vi "Timeout value.vi"(11 "Loop data in":T1={"Config"={"List"=[], "max rows"=8, "Listbox placement"=enum."None", "String Color Options"={"Use? (F)"=FALSE, "Color - Valid"=0, "Color - Invalid"=0, "Allow blank?"=FALSE}}, "Refs"={"String"=refnum, "Listbox"=refnum}, "State"={"LB active?"=FALSE}}) -> (3 "Loop data out":T1={"Config"={"List"=[], "max rows"=8, "Listbox placement"=enum."None", "String Color Options"={"Use? (F)"=FALSE, "Color - Valid"=0, "Color - Invalid"=0, "Allow blank?"=FALSE}}, "Refs"={"String"=refnum, "Listbox"=refnum}, "State"={"LB active?"=FALSE}}, 5 "timeout (ms)":i32)   [LabVIEW 2021, in "Autocomplete Textbox.lvlib"]
uses:
  Autocomplete Textbox.lvlib
  Loop Data.ctl
  Inputs.ctl
  Classes/Handle/Listbox placement.ctl
  Color String Options.ctl
  Refs.ctl
  State data.ctl
  Classes/Handle/Handle.lvclass
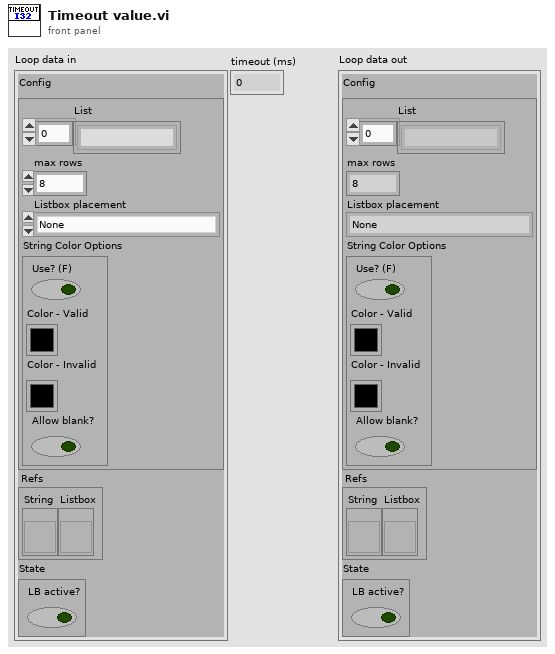
[diagram p1: front panel]
types:
  T1 = typedef "Autocomplete Textbox.lvlib/Loop Data.ctl" = cluster{"Config":T2, "Refs":T5, "State":T6}
  T2 = typedef "Autocomplete Textbox.lvlib/Inputs.ctl" = cluster{"List":string[], "max rows":i32, "Listbox placement":T3, "String Color Options":T4}
  T3 = typedef "Autocomplete Textbox.lvlib/Handle.lvclass/Listbox placement.ctl" = enum16{"None", "Under String", "Fit to Pane"}
  T4 = typedef "Autocomplete Textbox.lvlib/Color String Options.ctl" = cluster{"Use? (F)":bool, "Color - Valid":u32, "Color - Invalid":u32, "Allow blank?":bool}
  T5 = typedef "Autocomplete Textbox.lvlib/Refs.ctl" = cluster{"String":refnum<vi>, "Listbox":refnum<vi>}
  T6 = typedef "Autocomplete Textbox.lvlib/State data.ctl" = cluster{"LB active?":bool}
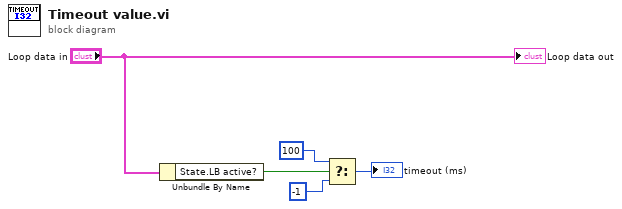
[diagram p0: block diagram]
diagram:
  n1 = Unbundle By Name("Loop data in") -> ("State.LB active?"=w4:bool)
  n2 = Select(t=100, s=w4, f=-1) -> (s? t:f=→"timeout (ms)":i32)
  "Loop data out" <- "Loop data in"
